vi "Save Config.vi"(8 "error in (no error)":errorcluster, 11 "Motion Controller in":refnum<class "Parent SIM Motion Controller.lvclass">) -> (0 "error out":errorcluster, 3 "Motion Controller out":refnum<class "Parent SIM Motion Controller.lvclass">)   [LabVIEW 2022 SP3, in "Parent SIM Motion Controller.lvclass"]
uses:
  Parent SIM Motion Controller.lvclass
  Parent SIM Motion Controller.lvclass/Parent SIM Motion Controller.ctl
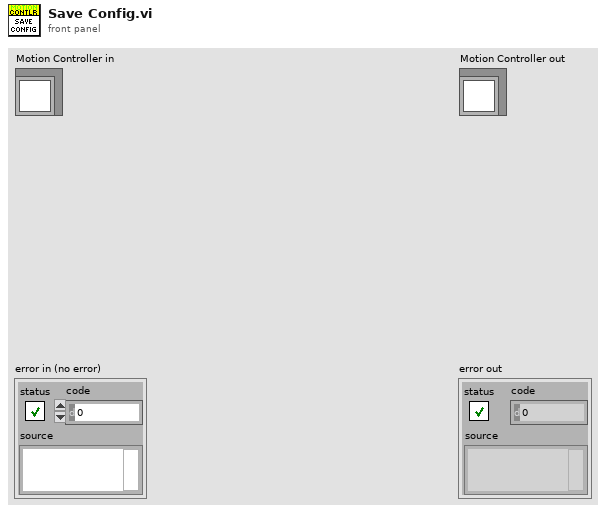
[diagram p1: front panel]
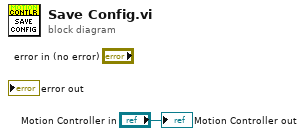
[diagram p0: block diagram]
diagram:
  "Motion Controller out" <- "Motion Controller in"
